vi "Roulette-Spin.vi"() -> ()   [LabVIEW 2019]
uses:
  <vilib>/Rock Robotics/WPI/ThirdParty/Phoenix-LabVIEW/Motor Controller/Controls/CTRE_Phoenix_MotorControl_ControlMode.ctl
  <vilib>/Rock Robotics/WPI/ThirdParty/Phoenix-LabVIEW/Motor Controller/Controls/CTRE_Phoenix_MotorControl_FeedbackDevice.ctl
  Robot Global Data.vi
  <vilib>/Rock Robotics/WPI/Utilities/WPI_GetSetVariantRefNum.vi
  <vilib>/Rock Robotics/WPI/ThirdParty/Phoenix-LabVIEW/Motor Controller/Get/CTRE_Phoenix_MotorController_GetSelectedSensorData.vi
panel:
  out "up":bool
  out "Position (Raw Sensor Units)":i32
  in  "F 2":dbl=0.0095 format="%#_13g"
  in  "D 2":dbl format="%#_13g"
  in  "I 2":dbl format="%#_13g"
  in  "P 2":dbl=0.5 format="%#_13g"
  in  "Max Acceleration 2":i32=2000
  in  "Cruise Velocity 2":i32=2000
  in  "Invalid Parmeter 2":dbl=63.0
  in  "F":dbl=0.0095 format="%#_13g"
  in  "D":dbl format="%#_13g"
  in  "I":dbl format="%#_13g"
  in  "P":dbl=0.5 format="%#_13g"
  in  "Max Acceleration":i32=15000
  in  "Cruise Velocity":i32=20000
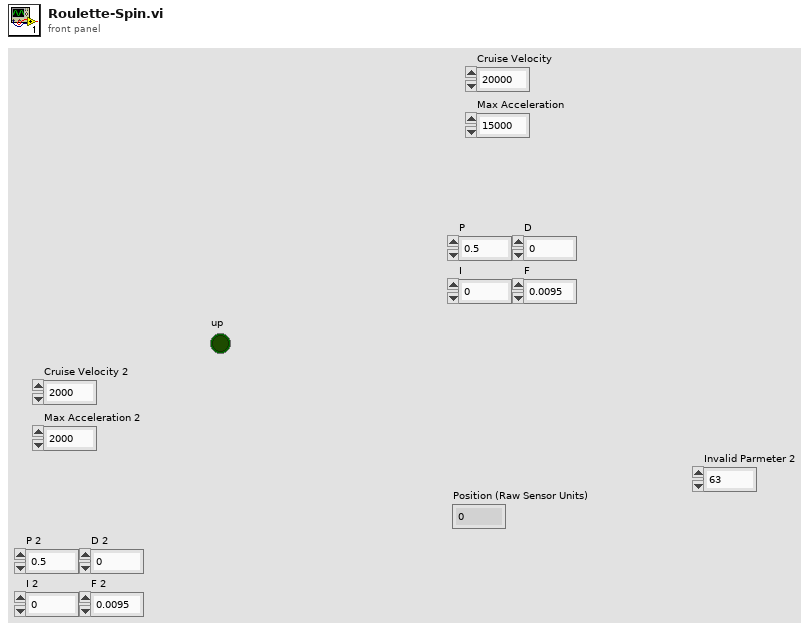
[diagram p1: front panel]
types:
  T1 = typedef "WPI_JoystickDevRef.ctl" = cluster{"Device":T2}
  T2 = typedef "WPI_JoystickDeviceEnum.ctl" = enum16{"USB 0", "USB 1", "USB 2", "USB 3", "USB 4", "USB 5"}
  T3 = typedef "WPI_MotorControlDeviceRef.ctl" = cluster{"DeviceStatus":errorcluster, "Type":T4, "PWM":cluster{"PWM Channel":T5, "DeadBand":T6}, "CAN":cluster{"Device Number":u8, "SetOutput VI Ref":variant, "GetOutput VI Ref":variant, "Enable VI Ref":variant, "Disable VI Ref":variant, "Data":variant}, "Invert":bool, "DIO PWM":cluster{"PWM \"Enable\" Channel":T5, "DIOChannel":T7, "PWM Rate":dbl}}
  T4 = typedef "WPI_MotorControlType.ctl" = enum16{"PWM", "CAN", "DIO PWM"}
  T5 = typedef "FPGA_DIOPWMChannel.ctl" = enum8{"PWM 0", "PWM 1", "PWM 2", "PWM 3", "PWM 4", "PWM 5", "PWM 6", "PWM 7", "PWM 8", "PWM 9", "PWM MXP 0", "PWM MXP 1", "PWM MXP 2", "PWM MXP 3", "PWM MXP 4", "PWM MXP 5", "PWM MXP 6", "PWM MXP 7", "PWM MXP 8", "PWM MXP 9", "Invalid"}
  T6 = typedef "WPI_PWMDeadband.ctl" = cluster{"Name":string, "maxPositivePwm":i32, "minPositivePwm":i32, "centerPwm":i32, "maxNegativePwm":i32, "minNegativePwm":i32, "angularRange":u16}
  T7 = typedef "FPGA_DIOChannel.ctl" = enum8{"DIO 0", "DIO 1", "DIO 2", "DIO 3", "DIO 4", "DIO 5", "DIO 6", "DIO 7", "DIO 8", "DIO 9", "DIO MXP 0", "DIO MXP 1", "DIO MXP 2", "DIO MXP 3", "DIO MXP 4", "DIO MXP 5", "DIO MXP 6", "DIO MXP 7", "DIO MXP 8", "DIO MXP 9", "DIO MXP 10", "DIO MXP 11", "DIO MXP 12", "DIO MXP 13", "DIO MXP 14", "DIO MXP 15", "SPI Port CS1", "SPI Port CS2", "SPI Port CS3", "SPI Port MISO", "SPI Port MOSI", "Invalid"}
  T8 = typedef "CTRE_Phoenix_MotorControl_ControlMode.ctl" = u16
  T9 = typedef "CTRE_Phoenix_MotorControl_FeedbackDevice.ctl" = i8
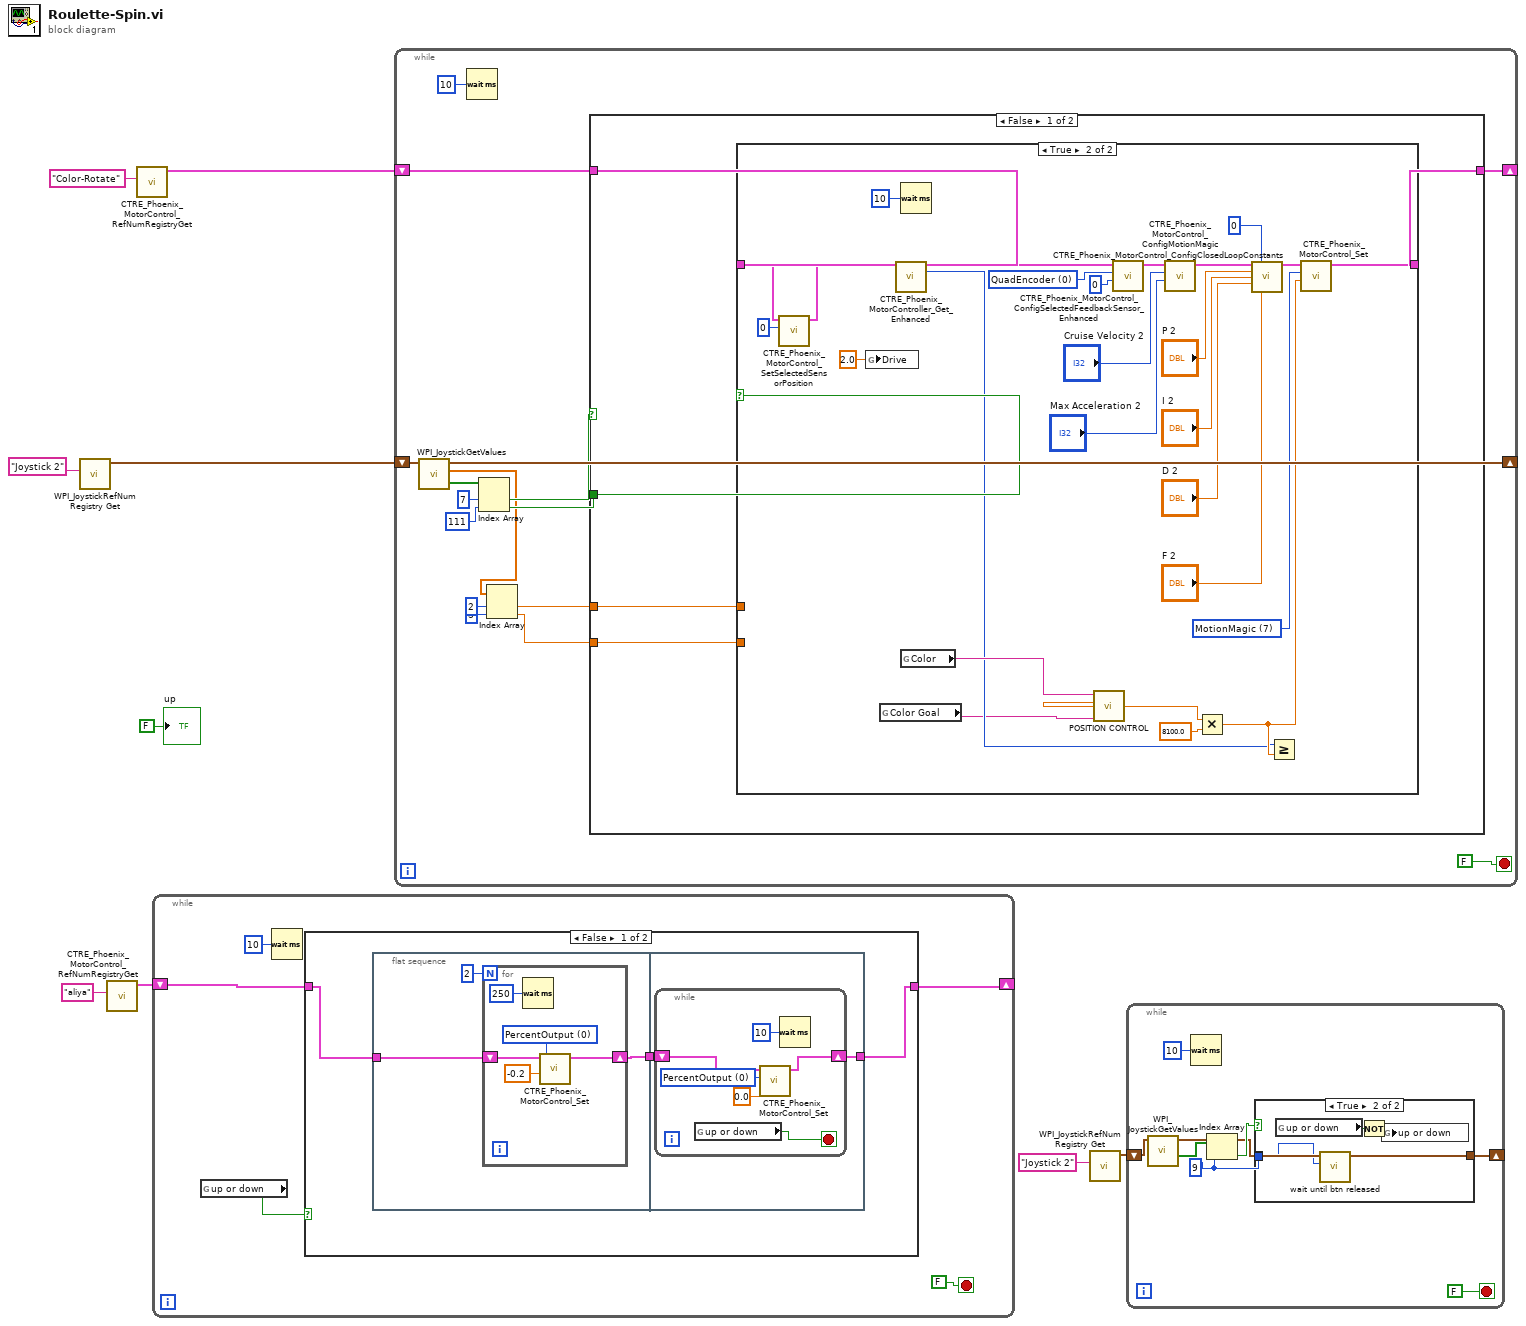
[diagram p0: block diagram]
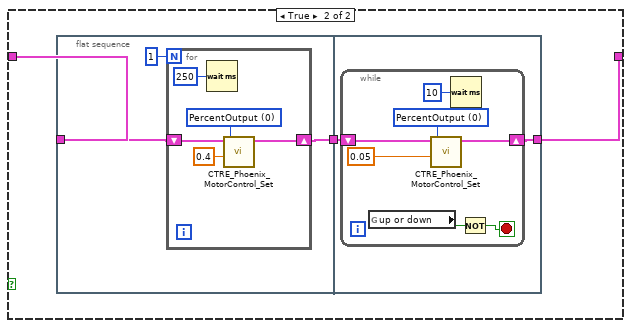
[diagram p3: hidden frame]
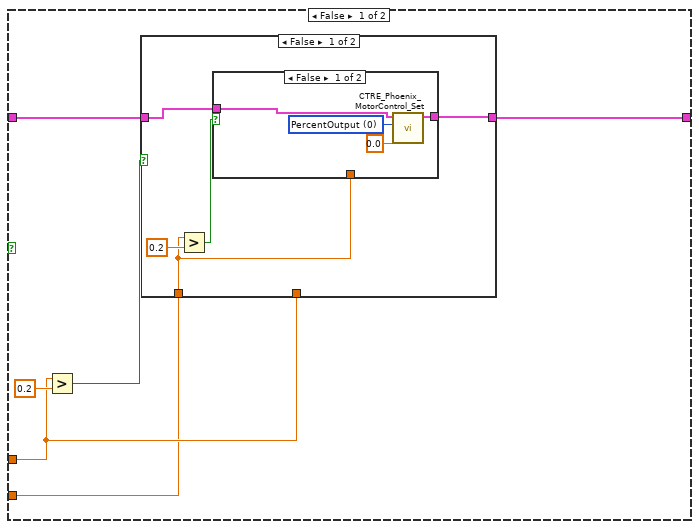
[diagram p4: hidden frame]
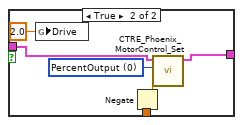
[diagram p5: hidden frame]
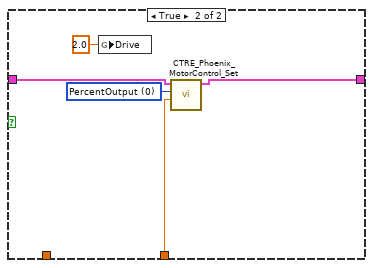
[diagram p6: hidden frame]
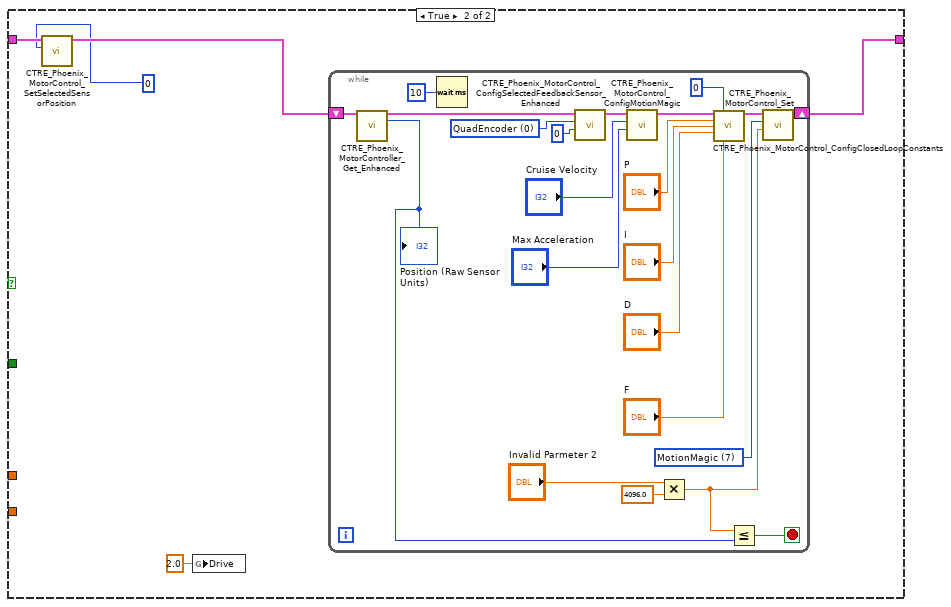
[diagram p7: hidden frame]
diagram:
  n1 = call <vilib>:"WPI_JoystickRefNum Registry Get.vi"("refnum name"="Joystick 2") -> ("JoystickDevRef"=w4:T1)  [unwired: 9 in, 1 out]
  n2 = call <vilib>:"CTRE_Phoenix_MotorControl_RefNumRegistryGet.vi"("refnum name"="aliya") -> ("PhoenixMotorControlDevRef"=w6:T3)  [unwired: 9 in, 1 out]
  n3 = call <vilib>:"CTRE_Phoenix_MotorControl_RefNumRegistryGet.vi"("refnum name"="Color-Rotate") -> ("PhoenixMotorControlDevRef"=w9:T3)  [unwired: 9 in, 1 out]
  n4 = while {
    shift-right: [w11] -> _
    shift-left: w6 -> [w12]
    stop <- FALSE stop-if-true
    n5 = global read "Robot Global Data.vi" "up or down"() -> (w10:bool)
    n6 = Wait (ms)(milliseconds to wait=u32 10) -> ()  [unwired: 1 out]
    n7 = case shown="False" w10 {
      tunnel: [w15 w35] -> w11
      tunnel: w12 -> [w16 w36]
      frame False {
        n8 = flat-sequence {
          tunnel: [w20] -> w17
          tunnel: w16 -> [w18]
          tunnel: [w26] -> w15
          tunnel: w17 -> [w27]
          frame #0 {
            n9 = for {
              N: 2 -> [_]
              shift-right: [w21] -> w20
              shift-left: w18 -> [w25]
              w23 = T8 0 items=["PercentOutput"=0, "Position"=1, "Velocity"=2, "Current"=3, "Follower"=5, "MotionProfile"=6, "MotionMagic"=7, "MotionProfileArc"=10, "Disabled"=15] ("Control Mode")
              n10 = Wait (ms)(milliseconds to wait=u32 250) -> ()  [unwired: 1 out]
              n11 = call <vilib>:"CTRE_Phoenix_MotorControl_Set.vi"("Output"=-0.2, "Control Mode"=w23, "PhoenixMotorControlDevRef"=w25) -> ("PhoenixMotorControlDevRef"=w21:T3)  [unwired: 7 in, 1 out]
            }
          }
          frame #1 {
            n12 = while {
              shift-right: [w32] -> w26
              shift-left: w27 -> [w33]
              stop <- w29 stop-if-true
              w31 = T8 0 items=["PercentOutput"=0, "Position"=1, "Velocity"=2, "Current"=3, "Follower"=5, "MotionProfile"=6, "MotionMagic"=7, "MotionProfileArc"=10, "Disabled"=15] ("Control Mode")
              n13 = global read "Robot Global Data.vi" "up or down"() -> (w29:bool)
              n14 = call <vilib>:"CTRE_Phoenix_MotorControl_Set.vi"("Output"=0.0, "Control Mode"=w31, "PhoenixMotorControlDevRef"=w33) -> ("PhoenixMotorControlDevRef"=w32:T3)  [unwired: 7 in, 1 out]
              n15 = Wait (ms)(milliseconds to wait=u32 10) -> ()  [unwired: 1 out]
            }
          }
        }
      }
      frame True {
        n16 = flat-sequence {
          tunnel: w36 -> [w39]
          tunnel: [w38] -> w34
          tunnel: [w46] -> w35
          tunnel: w34 -> [w45]
          frame #0 {
            n17 = for {
              N: 1 -> [_]
              shift-right: [w40] -> w38
              shift-left: w39 -> [w44]
              w42 = T8 0 items=["PercentOutput"=0, "Position"=1, "Velocity"=2, "Current"=3, "Follower"=5, "MotionProfile"=6, "MotionMagic"=7, "MotionProfileArc"=10, "Disabled"=15] ("Control Mode")
              n18 = Wait (ms)(milliseconds to wait=u32 250) -> ()  [unwired: 1 out]
              n19 = call <vilib>:"CTRE_Phoenix_MotorControl_Set.vi"("Output"=0.4, "Control Mode"=w42, "PhoenixMotorControlDevRef"=w44) -> ("PhoenixMotorControlDevRef"=w40:T3)  [unwired: 7 in, 1 out]
            }
          }
          frame #1 {
            n20 = while {
              shift-right: [w51] -> w46
              shift-left: w45 -> [w50]
              stop <- w49 stop-if-true
              w52 = T8 0 items=["PercentOutput"=0, "Position"=1, "Velocity"=2, "Current"=3, "Follower"=5, "MotionProfile"=6, "MotionMagic"=7, "MotionProfileArc"=10, "Disabled"=15] ("Control Mode")
              n21 = global read "Robot Global Data.vi" "up or down"() -> (w48:bool)
              n22 = call <vilib>:"CTRE_Phoenix_MotorControl_Set.vi"("Output"=0.05, "Control Mode"=w52, "PhoenixMotorControlDevRef"=w50) -> ("PhoenixMotorControlDevRef"=w51:T3)  [unwired: 7 in, 1 out]
              n23 = Wait (ms)(milliseconds to wait=u32 10) -> ()  [unwired: 1 out]
              n24 = Not(x=w48) -> (.not. x?=w49:bool)
            }
          }
        }
      }
    }
  }
  n25 = while {
    shift-right: [w68] -> _
    shift-left: w9 -> [w66]
    shift-right: [w62] -> _
    shift-left: w4 -> [w63]
    stop <- FALSE stop-if-true
    n26 = call <vilib>:"WPI_JoystickGetValues.vi"("JoystickDevRef"=w63) -> ("Buttons"=w64:bool[], "Axes"=w58:dbl[], "JoystickDevRef"=w62:T1)  [unwired: 6 in, 2 out]
    n27 = Wait (ms)(milliseconds to wait=u32 10) -> ()  [unwired: 1 out]
    n28 = Index Array(array=w64, index #1=7 ("index"), index #2=111 ("index")) -> (element #1=w61:bool, element #2=w59:bool)
    n29 = Index Array(array=w58, index #1=2 ("index"), index #2=3 ("index")) -> (element #1=w57:dbl, element #2=w56:dbl)
    n30 = case shown="False" w61 {
      tunnel: [w72 w131] -> w68
      tunnel: w66 -> [w73 w130]
      tunnel: w59 -> [w74 _]
      tunnel: w57 -> [w71 _]
      tunnel: w56 -> [w70 _]
      frame False {
        n31 = case shown="True" w74 {
          tunnel: w73 -> [w78 w125]
          tunnel: [w77 w126] -> w72
          tunnel: w71 -> [w76 _]
          tunnel: w70 -> [w75 _]
          frame False {
            n32 = Greater?(x=w76, y=0.2) -> (0:w79:bool)
            n33 = case shown="False" w79 {
              tunnel: w78 -> [w85 w100]
              tunnel: [w84 w99] -> w77
              tunnel: w76 -> [_ w97]
              tunnel: w75 -> [w81 _]
              frame False {
                n34 = Greater?(x=w81, y=0.2) -> (0:w82:bool)
                n35 = case shown="False" w82 {
                  tunnel: w85 -> [w87 w94]
                  tunnel: [w86 w93] -> w84
                  tunnel: w81 -> [_ w92]
                  frame False {
                    w89 = T8 0 items=["PercentOutput"=0, "Position"=1, "Velocity"=2, "Current"=3, "Follower"=5, "MotionProfile"=6, "MotionMagic"=7, "MotionProfileArc"=10, "Disabled"=15] ("Control Mode")
                    n36 = call <vilib>:"CTRE_Phoenix_MotorControl_Set.vi"("Output"=0.0, "Control Mode"=w89, "PhoenixMotorControlDevRef"=w87) -> ("PhoenixMotorControlDevRef"=w86:T3)  [unwired: 7 in, 1 out]
                  }
                  frame True {
                    w95 = T8 0 items=["PercentOutput"=0, "Position"=1, "Velocity"=2, "Current"=3, "Follower"=5, "MotionProfile"=6, "MotionMagic"=7, "MotionProfileArc"=10, "Disabled"=15] ("Control Mode")
                    n37 = global write "Robot Global Data.vi" "Drive"(2.0 ("Drive")) -> ()
                    n38 = Negate(x=w92) -> (-x=w91:dbl)
                    n39 = call <vilib>:"CTRE_Phoenix_MotorControl_Set.vi"("Output"=w91, "Control Mode"=w95, "PhoenixMotorControlDevRef"=w94) -> ("PhoenixMotorControlDevRef"=w93:T3)  [unwired: 7 in, 1 out]
                  }
                }
              }
              frame True {
                w98 = T8 0 items=["PercentOutput"=0, "Position"=1, "Velocity"=2, "Current"=3, "Follower"=5, "MotionProfile"=6, "MotionMagic"=7, "MotionProfileArc"=10, "Disabled"=15] ("Control Mode")
                n40 = global write "Robot Global Data.vi" "Drive"(2.0 ("Drive")) -> ()
                n41 = call <vilib>:"CTRE_Phoenix_MotorControl_Set.vi"("Output"=w97, "Control Mode"=w98, "PhoenixMotorControlDevRef"=w100) -> ("PhoenixMotorControlDevRef"=w99:T3)  [unwired: 7 in, 1 out]
              }
            }
          }
          frame True {
            w116 = T9 0 items=["None"=-1, "QuadEncoder"=0, "Analog"=2, "Tachometer"=4, "Pulse Width Encoded Position"=8, "Sensor Sum (S0 + S1)"=9, "Sensor Difference (D0 - D1)"=10, "Remote Source 0"=11, "Remote Source 1"=12, "Software Emulated"=15] ("Feedback Device")
            w122 = T8 7 items=["PercentOutput"=0, "Position"=1, "Velocity"=2, "Follower"=5, "MotionProfile"=6, "MotionMagic"=7, "MotionMagicArc"=8, "TimedPercentOutput"=9, "Disabled"=15] ("Control Mode")
            n42 = call <vilib>:"CTRE_Phoenix_MotorControl_SetSelectedSensorPosition.vi"("New Sensor Position"=0, "PhoenixMotorControlDevRef"=w125) -> ("PhoenixMotorControlDevRef"=w124:T3)  [unwired: 8 in, 1 out]
            n43 = global write "Robot Global Data.vi" "Drive"(2.0 ("Drive")) -> ()
            n44 = global read "Robot Global Data.vi" "Color Goal"() -> (w102:string)
            n45 = call-poly <vilib>:"CTRE_Phoenix_MotorController_Get_Enhanced.vi"("PhoenixMotorControlDevRef"=w124) -> ("PhoenixMotorControlDevRef"=w104:T3, "Position (Raw Sensor Units)"=w103:i32)  [unwired: 11 in, 2 out]
            n46 = Wait (ms)(milliseconds to wait=u32 10) -> ()  [unwired: 1 out]
            n47 = global read "Robot Global Data.vi" "Color"() -> (w119:string)
            n48 = call "POSITION CONTROL.vi"("Goal"=w102, "Current Color"=w119) -> ("Result"=w120:dbl)  [unwired: 9 in]
            n49 = call <vilib>:"CTRE_Phoenix_MotorControl_ConfigSelectedFeedbackSensor_Enhanced.vi"("pidLoopIdx"=0, "Feedback Device"=w116, "PhoenixMotorControlDevRef"=w104) -> ("PhoenixMotorControlDevRef"=w115:T3)  [unwired: 7 in, 1 out]
            n50 = call <vilib>:"CTRE_Phoenix_MotorControl_ConfigMotionMagic.vi"("Acceleration"="Max Acceleration 2", "Cruise Velocity"="Cruise Velocity 2", "PhoenixMotorControlDevRef"=w115) -> ("PhoenixMotorControlDevRef"=w112:T3)  [unwired: 7 in, 1 out]
            n51 = Multiply(x=w120, y=8100.0) -> (x*y=w117:dbl)
            n52 = call <vilib>:"CTRE_Phoenix_MotorControl_ConfigClosedLoopConstants.vi"("PhoenixMotorControlDevRef"=w112, "slotIdx"=0, "P"="P 2", "I"="I 2", "D"="D 2", "F"="F 2") -> ("PhoenixMotorControlDevRef"=w105:T3)  [unwired: 8 in, 1 out]
            n53 = Greater Or Equal?(x=w103, y=w117) -> ()  [unwired: 1 out]
            n54 = call <vilib>:"CTRE_Phoenix_MotorControl_Set.vi"("Output"=w117, "Control Mode"=w122, "PhoenixMotorControlDevRef"=w105) -> ("PhoenixMotorControlDevRef"=w126:T3)  [unwired: 7 in, 1 out]
          }
        }
      }
      frame True {
        n55 = call <vilib>:"CTRE_Phoenix_MotorControl_SetSelectedSensorPosition.vi"("New Sensor Position"=0, "PhoenixMotorControlDevRef"=w130) -> ("PhoenixMotorControlDevRef"=w129:T3)  [unwired: 8 in, 1 out]
        n56 = global write "Robot Global Data.vi" "Drive"(2.0 ("Drive")) -> ()
        n57 = while {
          shift-right: [w153] -> w131
          shift-left: w129 -> [w152]
          stop <- w132 stop-if-true
          w140 = T8 7 items=["PercentOutput"=0, "Position"=1, "Velocity"=2, "Follower"=5, "MotionProfile"=6, "MotionMagic"=7, "MotionMagicArc"=8, "TimedPercentOutput"=9, "Disabled"=15] ("Control Mode")
          w151 = T9 0 items=["None"=-1, "QuadEncoder"=0, "Analog"=2, "Tachometer"=4, "Pulse Width Encoded Position"=8, "Sensor Sum (S0 + S1)"=9, "Sensor Difference (D0 - D1)"=10, "Remote Source 0"=11, "Remote Source 1"=12, "Software Emulated"=15] ("Feedback Device")
          n58 = call-poly <vilib>:"CTRE_Phoenix_MotorController_Get_Enhanced.vi"("PhoenixMotorControlDevRef"=w152) -> ("PhoenixMotorControlDevRef"=w136:T3, "Position (Raw Sensor Units)"=w133:i32)  [unwired: 11 in, 2 out]
          "Position (Raw Sensor Units)" <- w133
          n59 = Wait (ms)(milliseconds to wait=u32 10) -> ()  [unwired: 1 out]
          n60 = call <vilib>:"CTRE_Phoenix_MotorControl_ConfigSelectedFeedbackSensor_Enhanced.vi"("pidLoopIdx"=0, "Feedback Device"=w151, "PhoenixMotorControlDevRef"=w136) -> ("PhoenixMotorControlDevRef"=w150:T3)  [unwired: 7 in, 1 out]
          n61 = call <vilib>:"CTRE_Phoenix_MotorControl_ConfigMotionMagic.vi"("Acceleration"="Max Acceleration", "Cruise Velocity"="Cruise Velocity", "PhoenixMotorControlDevRef"=w150) -> ("PhoenixMotorControlDevRef"=w147:T3)  [unwired: 7 in, 1 out]
          n62 = Multiply(x="Invalid Parmeter 2", y=4096.0) -> (x*y=w134:dbl)
          n63 = call <vilib>:"CTRE_Phoenix_MotorControl_ConfigClosedLoopConstants.vi"("PhoenixMotorControlDevRef"=w147, "slotIdx"=0, "P"="P", "I"="I", "D"="D", "F"="F") -> ("PhoenixMotorControlDevRef"=w139:T3)  [unwired: 8 in, 1 out]
          n64 = Less Or Equal?(x=w134, y=w133) -> (x <= y?=w132:bool)
          n65 = call <vilib>:"CTRE_Phoenix_MotorControl_Set.vi"("Output"=w134, "Control Mode"=w140, "PhoenixMotorControlDevRef"=w139) -> ("PhoenixMotorControlDevRef"=w153:T3)  [unwired: 7 in, 1 out]
        }
      }
    }
  }
  n66 = call <vilib>:"WPI_JoystickRefNum Registry Get.vi"("refnum name"="Joystick 2") -> ("JoystickDevRef"=w1:T1)  [unwired: 9 in, 1 out]
  n67 = while {
    shift-right: [w156] -> _
    shift-left: w1 -> [w157]
    stop <- FALSE stop-if-true
    w158 = 9 ("index")
    n68 = call <vilib>:"WPI_JoystickGetValues.vi"("JoystickDevRef"=w157) -> ("Buttons"=w161:bool[], "JoystickDevRef"=w159:T1)  [unwired: 6 in, 3 out]
    n69 = Wait (ms)(milliseconds to wait=u32 10) -> ()  [unwired: 1 out]
    n70 = Index Array(array=w161, index=w158) -> (element=w160:bool)
    n71 = case shown="True" w160 {
      tunnel: w159 -> [w162 w167]
      tunnel: [w162 w166] -> w156
      tunnel: w158 -> [_ w165]
      frame False {
      }
      frame True {
        n72 = global read "Robot Global Data.vi" "up or down"() -> (w164:bool)
        n73 = call "wait until btn released.vi"("index"=w165, "JoystickDevRef"=w167) -> ("JoystickDevRef 2"=w166:T1)  [unwired: 9 in]
        n74 = Not(x=w164) -> (.not. x?=w163:bool)
        n75 = global write "Robot Global Data.vi" "up or down"(w163) -> ()
      }
    }
  }
  "up" <- FALSE ("up")
